vi "Publicador2.vi"() -> ()   [LabVIEW 2018]
uses:
  RxTx/RxTx.lvclass
  <vilib>/addons/zeromq/zmq_context.lvclass
  socket REP/socket REP.lvclass
  C:/Users/Denis/Desktop/communication-manager/communication-manager/Socket/Socket.lvclass
  socket PUB/socket PUB.lvclass
  Socket/Socket.lvclass
panel:
  in  "socket PUB.lvclass":refnum<class "socket PUB.lvclass">
  in  "socket REP.lvclass":refnum<class "socket REP.lvclass">
  out "error out 2":errorcluster
  out "context":refnum<class "zmq_context.lvclass">
  in  "Queue RX":refnum<class "RxTx.lvclass">
  in  "Comm Type":string(combo)="REP"
  out "Request":string
  in  "stop":bool
  # "REP/PUB endpoint"
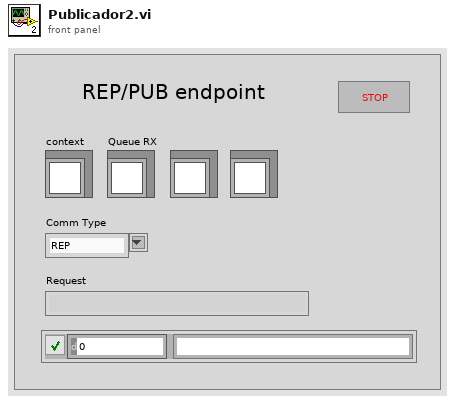
[diagram p1: front panel]
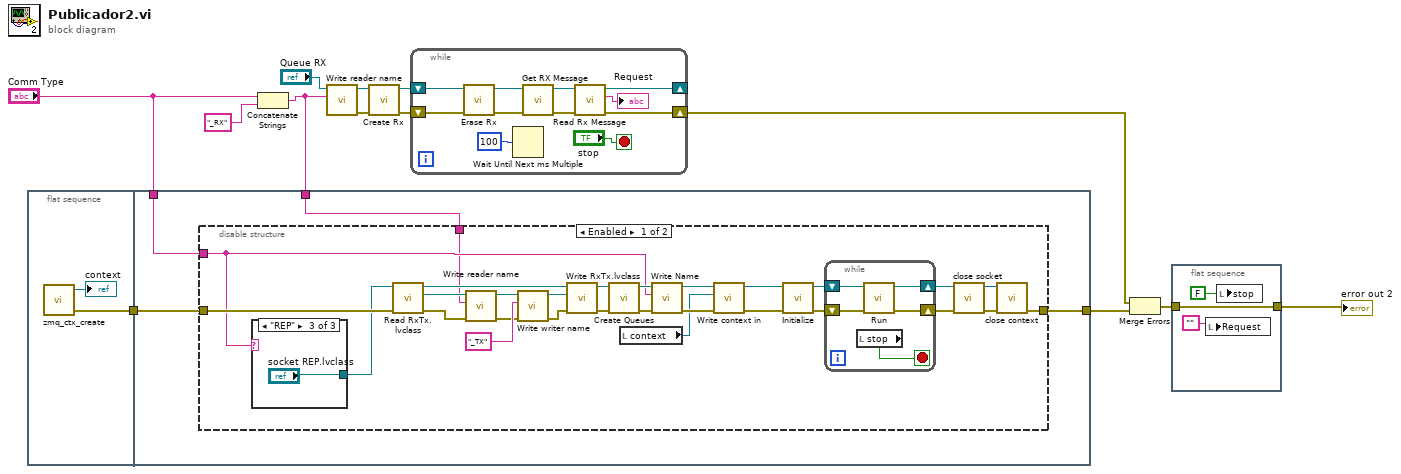
[diagram p0: block diagram]
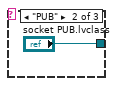
[diagram p3: hidden frame]
diagram:
  n1 = flat-sequence {
    tunnel: [w14] -> w5
    tunnel: [w19] -> w7
    tunnel: w5 -> [w18]
    tunnel: "Comm Type" -> [w17]
    tunnel: w1 -> [w16]
    frame #0 {
      n2 = call <vilib>:"zmq_ctx_create.vi"() -> ("error out"=w14:errorcluster, "context out"=→"context":refnum<class "zmq_context.lvclass">)  [unwired: 4 in]
    }
    frame #1 {
      n3 = disable-structure shown="Enabled" {
        disable-tunnel: [w24 _] -> w19
        disable-tunnel: w18 -> [w23 _]
        disable-tunnel: w17 -> [w22 _]
        disable-tunnel: w16 -> [w20 _]
        frame Enabled {
          n4 = case shown="\"REP\"" w22 {
            tunnel: [_ "socket PUB.lvclass" "socket REP.lvclass"] -> w21
            frame "False", Default {
            }
            frame "PUB" {
            }
            frame "REP" {
            }
          }
          n5 = call-dynamic "Read RxTx.lvclass.vi"("error in (no error)"=w23, "Socket in"=w21) -> ("error out"=w40:errorcluster, "RxTx.lvclass"=w46:refnum<class "RxTx.lvclass">, "Socket out"=w43:refnum<class "Socket.lvclass">)  [unwired: 7 in]
          n6 = call-dynamic "Write reader name.vi"("error in (no error)"=w40, "RX name"=w20, "RxTx in"=w46) -> ("error out"=w39:errorcluster, "RxTx out"=w45:refnum<class "RxTx.lvclass">)  [unwired: 7 in]
          n7 = call-dynamic "Write writer name.vi"("error in (no error)"=w39, "Tx name"="_TX" ("writer name"), "RxTx in"=w45) -> ("error out"=w38:errorcluster, "RxTx out"=w44:refnum<class "RxTx.lvclass">)  [unwired: 7 in]
          n8 = call-dynamic "Write RxTx.lvclass.vi"("error in (no error)"=w38, "RxTx.lvclass"=w44, "Socket in"=w43) -> ("error out"=w41:errorcluster, "Socket out"=w42:refnum<class "Socket.lvclass">)  [unwired: 7 in]
          n9 = call-dynamic "Create Queues.vi"("error in (no error)"=w41, "Socket in"=w42) -> ("error out"=w34:errorcluster, "Socket out"=w37:refnum<class "Socket.lvclass">)  [unwired: 8 in]
          n10 = local read "context"() -> (w27:refnum<class "zmq_context.lvclass">)
          n11 = call-dynamic "Write Name.vi"("error in (no error)"=w34, "Name"=w22, "Socket in"=w37) -> ("error out"=w33:errorcluster, "Socket out"=w36:refnum<class "Socket.lvclass">)  [unwired: 7 in]
          n12 = call-dynamic "Write context in.vi"("error in (no error)"=w33, "zeromq.lvlib:ZeroMQ Context"=w27, "Socket in"=w36) -> ("error out"=w32:errorcluster, "Socket out"=w35:refnum<class "Socket.lvclass">)  [unwired: 7 in]
          n13 = call-dynamic "Initialize.vi"("error in (no error)"=w32, "Socket in"=w35) -> ("error out"=w29:errorcluster, "Socket out"=w31:refnum<class "Socket.lvclass">)  [unwired: 8 in]
          n14 = while {
            shift-right: [w53] -> w30
            shift-left: w31 -> [w54]
            shift-right: [w51] -> w28
            shift-left: w29 -> [w52]
            stop <- w50 stop-if-true
            n15 = local read "stop"() -> (w50:bool)
            n16 = call-dynamic "Run.vi"("error in (no error)"=w52, "Socket in"=w54) -> ("error out"=w51:errorcluster, "Socket out"=w53:refnum<class "Socket.lvclass">)  [unwired: 8 in]
          }
          n17 = call "close socket.vi"("error in (no error)"=w28, "Socket in"=w30) -> ("error out"=w26:errorcluster, "Socket out"=w25:refnum<class "Socket.lvclass">)  [unwired: 8 in]
          n18 = call-dynamic "close context.vi"("error in (no error)"=w26, "Socket in"=w25) -> ("error out"=w24:errorcluster)  [unwired: 8 in, 1 out]
        }
        frame Disabled {
        }
      }
    }
  }
  n19 = Concatenate Strings("Comm Type", "_RX" ("string")) -> (w1:string)
  n20 = call-dynamic "Write reader name.vi"("RX name"=w1, "RxTx in"="Queue RX") -> ("error out"=w10:errorcluster, "RxTx out"=w11:refnum<class "RxTx.lvclass">)  [unwired: 8 in]
  n21 = call "Create Rx.vi"("error in (no error)"=w10, "RxTx in"=w11) -> ("error out"=w9:errorcluster, "RxTx out"=w13:refnum<class "RxTx.lvclass">)  [unwired: 8 in]
  n22 = while {
    shift-right: [w63] -> _
    shift-left: w13 -> [w56]
    shift-right: [w60] -> w8
    shift-left: w9 -> [w59]
    stop <- "stop" stop-if-true
    n23 = call "Erase Rx.vi"("error in (no error)"=w59, "RxTx in"=w56) -> ("error out"=w58:errorcluster, "RxTx out"=w57:refnum<class "RxTx.lvclass">)  [unwired: 8 in]
    n24 = Wait Until Next ms Multiple(millisecond multiple=u32 100) -> ()  [unwired: 1 out]
    n25 = call "Get RX Message.vi"("error in (no error)"=w58, "RxTx in"=w57) -> ("error out"=w61:errorcluster, "RxTx out"=w64:refnum<class "RxTx.lvclass">)  [unwired: 7 in, 1 out]
    n26 = call "Read Rx Message.vi"("error in (no error)"=w61, "RxTx in"=w64) -> ("error out"=w60:errorcluster, "Rx Message"=→"Request":string, "RxTx out"=w63:refnum<class "RxTx.lvclass">)  [unwired: 7 in]
  }
  n27 = Merge Errors(w8, w7) -> (w6:errorcluster)
  n28 = flat-sequence {
    tunnel: w6 -> [w68]
    tunnel: [w68] -> w4
    frame #0 {
      n29 = local write "Request"("") -> ()
      n30 = local write "stop"(FALSE ("stop")) -> ()
    }
  }
  "error out 2" <- w4
